vi "Trigger_Loggic.vi"(8 "error in (no error)":errorcluster) -> (0 "error out":errorcluster, 3 "Array":i32[](array[numeric]))   [LabVIEW 2017]
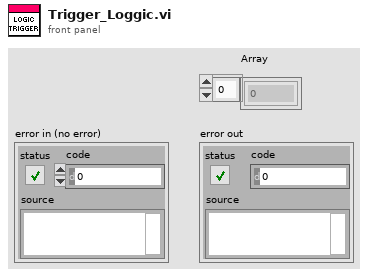
[diagram p1: front panel]
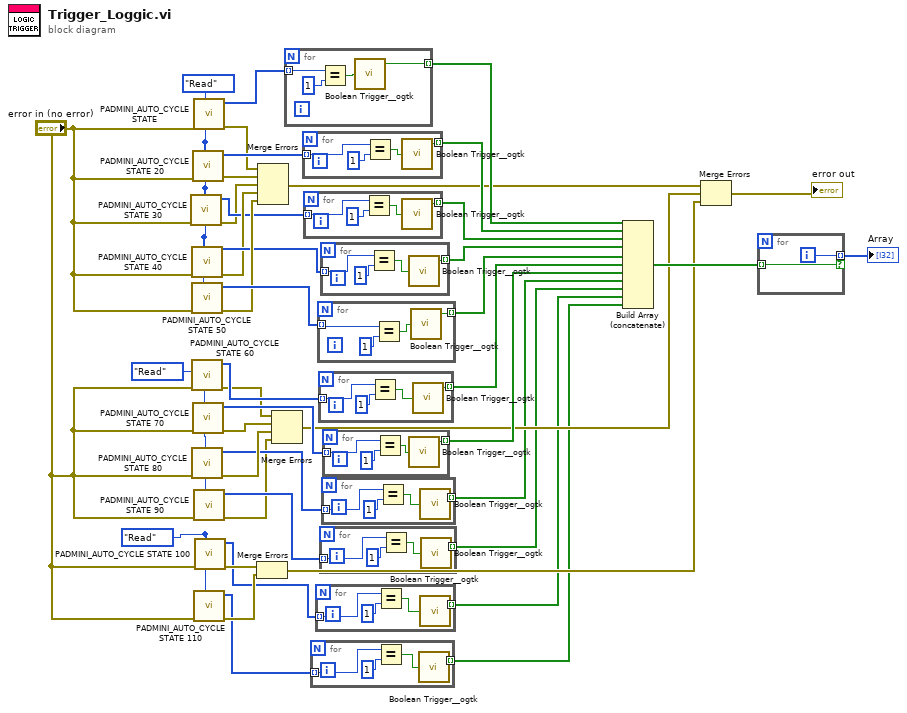
[diagram p0: block diagram]
diagram:
  w1 = enum16{"Read", "Write"}."Read" ("Enum")
  w2 = enum16{"Read", "Write"}."Read" ("Enum")
  w5 = enum16{"Read", "Write"}."Read" ("Enum")
  n1 = call "PADMINI_AUTO_CYCLE STATE 30.vi"("Enum"=w5, "error in (no error)"="error in (no error)") -> ("error out"=w31:errorcluster, "Input 2"=w32:i32[])  [unwired: 8 in]
  n2 = call "PADMINI_AUTO_CYCLE STATE 40.vi"("Enum"=w5, "error in (no error)"="error in (no error)") -> ("error out"=w34:errorcluster, "Input 2"=w35:i32[])  [unwired: 8 in]
  n3 = call "PADMINI_AUTO_CYCLE STATE 50.vi"("Enum"=w5, "error in (no error)"="error in (no error)") -> ("error out"=w37:errorcluster, "Input 2"=w38:i32[])  [unwired: 8 in]
  n4 = call "PADMINI_AUTO_CYCLE STATE 60.vi"("Enum"=w2, "error in (no error)"="error in (no error)") -> ("error out"=w22:errorcluster, "Input 2"=w40:i32[])  [unwired: 8 in]
  n5 = call "PADMINI_AUTO_CYCLE STATE 80.vi"("Enum"=w2, "error in (no error)"="error in (no error)") -> ("error out"=w17:errorcluster, "Input 2"=w16:i32[])  [unwired: 8 in]
  n6 = call "PADMINI_AUTO_CYCLE STATE 20.vi"("Enum"=w5, "error in (no error)"="error in (no error)") -> ("error out"=w25:errorcluster, "Input 2"=w27:i32[])  [unwired: 8 in]
  n7 = call "PADMINI_AUTO_CYCLE STATE 70.vi"("Enum"=w2, "error in (no error)"="error in (no error)") -> ("error out"=w21:errorcluster, "Input 2"=w42:i32[])  [unwired: 8 in]
  n8 = call "PADMINI_AUTO_CYCLE STATE.vi"("Enum"=w5, "error in (no error)"="error in (no error)") -> ("error out"=w26:errorcluster, "Input 2"=w29:i32[])  [unwired: 8 in]
  n9 = call "PADMINI_AUTO_CYCLE STATE 90.vi"("Enum"=w2, "error in (no error)"="error in (no error)") -> ("error out"=w11:errorcluster, "Input 2"=w14:i32[])  [unwired: 8 in]
  n10 = call "PADMINI_AUTO_CYCLE STATE 110.vi"("Enum"=w1, "error in (no error)"="error in (no error)") -> ("error out"=w10:errorcluster, "Input 2"=w6:i32[])  [unwired: 8 in]
  n11 = call "PADMINI_AUTO_CYCLE STATE 100.vi"("Enum"=w1, "error in (no error)"="error in (no error)") -> ("error out"=w9:errorcluster, "Input 2"=w7:i32[])  [unwired: 8 in]
  n12 = Merge Errors(w9, w10) -> (w8:errorcluster)
  n13 = Merge Errors(w26, w25, w31, w34, w37) -> (w19:errorcluster)
  n14 = Merge Errors(w22, w21, w17, w11) -> (w20:errorcluster)
  n15 = for {
    tunnel: w29 -> [w46] mode=indexing
    tunnel: [w47] -> w30 mode=indexing
    n16 = Equal?(x=w46, y=1) -> (x = y?=w44:bool)
    n17 = call <userlib>:"Boolean Trigger__ogtk.vi"("Boolean Input"=w44) -> ("Rising Edge"=w47:bool)  [unwired: 1 in, 1 out]
  }
  n18 = for {
    tunnel: w27 -> [w50] mode=indexing
    tunnel: [w51] -> w28 mode=indexing
    n19 = Equal?(x=w50, y=1) -> (x = y?=w49:bool)
    n20 = call <userlib>:"Boolean Trigger__ogtk.vi"("Boolean Input"=w49) -> ("Rising Edge"=w51:bool)  [unwired: 1 in, 1 out]
  }
  n21 = for {
    tunnel: w32 -> [w52] mode=indexing
    tunnel: [w55] -> w33 mode=indexing
    n22 = Equal?(x=w52, y=1) -> (x = y?=w53:bool)
    n23 = call <userlib>:"Boolean Trigger__ogtk.vi"("Boolean Input"=w53) -> ("Rising Edge"=w55:bool)  [unwired: 1 in, 1 out]
  }
  n24 = for {
    tunnel: w6 -> [w56] mode=indexing
    tunnel: [w59] -> w3 mode=indexing
    n25 = Equal?(x=w56, y=1) -> (x = y?=w57:bool)
    n26 = call <userlib>:"Boolean Trigger__ogtk.vi"("Boolean Input"=w57) -> ("Rising Edge"=w59:bool)  [unwired: 1 in, 1 out]
  }
  n27 = for {
    tunnel: w7 -> [w60] mode=indexing
    tunnel: [w63] -> w4 mode=indexing
    n28 = Equal?(x=w60, y=1) -> (x = y?=w61:bool)
    n29 = call <userlib>:"Boolean Trigger__ogtk.vi"("Boolean Input"=w61) -> ("Rising Edge"=w63:bool)  [unwired: 1 in, 1 out]
  }
  n30 = for {
    tunnel: w38 -> [w64] mode=indexing
    tunnel: [w67] -> w39 mode=indexing
    n31 = Equal?(x=w64, y=1) -> (x = y?=w65:bool)
    n32 = call <userlib>:"Boolean Trigger__ogtk.vi"("Boolean Input"=w65) -> ("Rising Edge"=w67:bool)  [unwired: 1 in, 1 out]
  }
  n33 = for {
    tunnel: w40 -> [w68] mode=indexing
    tunnel: [w71] -> w41 mode=indexing
    n34 = Equal?(x=w68, y=1) -> (x = y?=w69:bool)
    n35 = call <userlib>:"Boolean Trigger__ogtk.vi"("Boolean Input"=w69) -> ("Rising Edge"=w71:bool)  [unwired: 1 in, 1 out]
  }
  n36 = for {
    tunnel: w14 -> [w72] mode=indexing
    tunnel: [w75] -> w13 mode=indexing
    n37 = Equal?(x=w72, y=1) -> (x = y?=w73:bool)
    n38 = call <userlib>:"Boolean Trigger__ogtk.vi"("Boolean Input"=w73) -> ("Rising Edge"=w75:bool)  [unwired: 1 in, 1 out]
  }
  n39 = for {
    tunnel: w35 -> [w76] mode=indexing
    tunnel: [w79] -> w36 mode=indexing
    n40 = Equal?(x=w76, y=1) -> (x = y?=w77:bool)
    n41 = call <userlib>:"Boolean Trigger__ogtk.vi"("Boolean Input"=w77) -> ("Rising Edge"=w79:bool)  [unwired: 1 in, 1 out]
  }
  n42 = for {
    tunnel: w16 -> [w80] mode=indexing
    tunnel: [w83] -> w15 mode=indexing
    n43 = Equal?(x=w80, y=1) -> (x = y?=w81:bool)
    n44 = call <userlib>:"Boolean Trigger__ogtk.vi"("Boolean Input"=w81) -> ("Rising Edge"=w83:bool)  [unwired: 1 in, 1 out]
  }
  n45 = for {
    tunnel: w42 -> [w84] mode=indexing
    tunnel: [w87] -> w43 mode=indexing
    n46 = Equal?(x=w84, y=1) -> (x = y?=w85:bool)
    n47 = call <userlib>:"Boolean Trigger__ogtk.vi"("Boolean Input"=w85) -> ("Rising Edge"=w87:bool)  [unwired: 1 in, 1 out]
  }
  n48 = Build Array (concatenate)(w30, w28, w33, w36, w39, w41, w43, w15, w13, w4, w3) -> (w24:bool[])
  n49 = Merge Errors(w19, w20, w8) -> (→"error out":errorcluster)
  n50 = for {
    tunnel: w24 -> [w88] mode=indexing
    tunnel: [w89] -> w23 mode=indexing if=w88
    i -> [w89]
  }
  "Array" <- w23
